vi "FileSync.FIFO, Sync Log.vi"(7 "MaxLen":i32=1000, 10 "New Event":T1, 11 "Array In":T1[](array[typedef])) -> (2 "Full":bool, 3 "Array Out":T1[](array[typedef]))   [LabVIEW 2024, in "KATE_Lib.lvlib" / "File Utils.lvlib" / "File.Sync.lvclass"]
uses:
  File.Sync.lvclass
  File.Sync Item Log Record.ctl
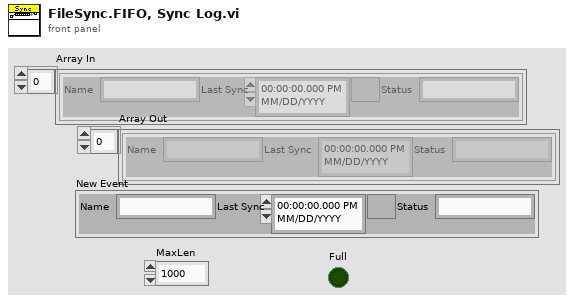
[diagram p1: front panel]
types:
  T1 = typedef "KATE_Lib.lvlib/File Utils.lvlib/File.Sync.lvclass/File.Sync Item Log Record.ctl" = cluster{"Name":string, "Last Sync":timestamp, "Status":string}
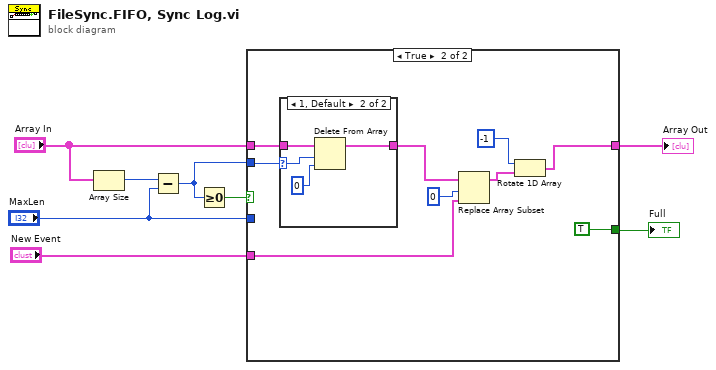
[diagram p0: block diagram]
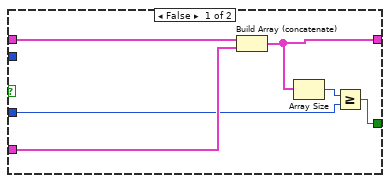
[diagram p2: hidden frame]
diagram:
  n1 = Array Size(array="Array In") -> (size(s)=w3:i32)
  n2 = Subtract(x=w3, y="MaxLen") -> (x-y=w5:i32)
  n3 = Greater Or Equal To 0?(x=w5) -> (x >= 0?=w4:bool)
  n4 = case shown="True" w4 {
    tunnel: "New Event" -> [w13 w22]
    tunnel: "Array In" -> [w14 w17]
    tunnel: [w12 w23] -> w8
    tunnel: w5 -> [_ w18]
    tunnel: [w9 TRUE] -> w1
    tunnel: "MaxLen" -> [w10 _]
    frame False {
      n5 = Build Array (concatenate)(w14, w13) -> (w12:T1[])
      n6 = Array Size(array=w12) -> (size(s)=w11:i32)
      n7 = Greater Or Equal?(x=w11, y=w10) -> (x >= y?=w9:bool)
    }
    frame True {
      n8 = case shown="1, Default" w18 {
        selector: w18 -> [_ w27]
        tunnel: w17 -> [w24 w28]
        tunnel: [w24 w26] -> w16
        frame 0 {
        }
        frame 1, Default {
          n9 = Delete From Array(array=w28, length=w27, index=0) -> (array with subset deleted=w26:T1[])  [unwired: 1 out]
        }
      }
      n10 = Replace Array Subset(array=w16, new element=w22, index=0) -> (w20:T1[])
      n11 = Rotate 1D Array(1:w20, 2:-1 ("index")) -> (0:w23:T1[])
    }
  }
  "Full" <- w1
  "Array Out" <- w8
